vi "Running Average.vi"(6 "Load Data":bool, 7 "Iteration Count In":i32, 8 "DSA Measurements In":sgl[][](array[numeric]), 9 "WT1800 Measurements In":sgl[][](array[numeric]), 10 "DSA Averages In":sgl[][](array[numeric]), 11 "WT1800 Averages In":sgl[][](array[numeric])) -> (2 "DSA Averages Out":sgl[][](array[numeric]), 3 "WT1800 Averages Out":sgl[][](array[numeric]), 5 "Iteration Count Out":i32)   [LabVIEW 2021]
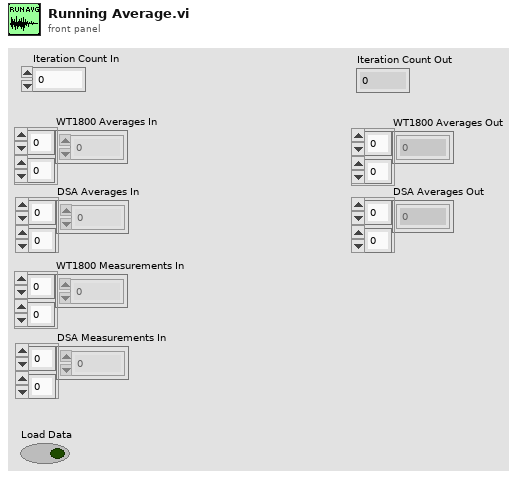
[diagram p1: front panel]
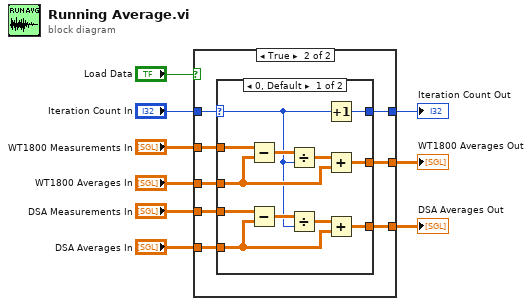
[diagram p0: block diagram]
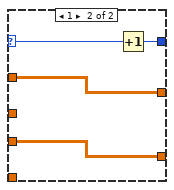
[diagram p3: hidden frame]
diagram:
  n1 = case shown="True" "Load Data" {
    tunnel: [w11 w18] -> w8
    tunnel: "WT1800 Measurements In" -> [_ w20]
    tunnel: "WT1800 Averages In" -> [w11 w19]
    tunnel: [w10 w17] -> w4
    tunnel: "DSA Measurements In" -> [_ w15]
    tunnel: "DSA Averages In" -> [w10 w16]
    tunnel: "Iteration Count In" -> [w12 w13]
    tunnel: [w12 w14] -> w2
    frame False {
    }
    frame True {
      n2 = case shown="0, Default" w13 {
        selector: w13 -> [w21 w34]
        tunnel: w20 -> [w31 w35]
        tunnel: w19 -> [w30 _]
        tunnel: [w28 w35] -> w18
        tunnel: [w27 w36] -> w17
        tunnel: w16 -> [w25 _]
        tunnel: w15 -> [w24 w36]
        tunnel: [w22 w33] -> w14
        frame 0, Default {
          n3 = Subtract(x=w31, y=w30) -> (x-y=w32:sgl[][])
          n4 = Subtract(x=w24, y=w25) -> (x-y=w23:sgl[][])
          n5 = Divide(x=w32, y=w21) -> (x/y=w29:sgl[][])
          n6 = Divide(x=w23, y=w21) -> (x/y=w26:sgl[][])
          n7 = Increment(x=w21) -> (x+1=w22:i32)
          n8 = Add(x=w29, y=w30) -> (x+y=w28:sgl[][])
          n9 = Add(x=w26, y=w25) -> (x+y=w27:sgl[][])
        }
        frame 1 {
          n10 = Increment(x=w34) -> (x+1=w33:i32)
        }
      }
    }
  }
  "WT1800 Averages Out" <- w8
  "DSA Averages Out" <- w4
  "Iteration Count Out" <- w2
